vi "JWT Calculate Hash.vi"(0 "JSONWebToken in":refnum<class "JSONWebToken.lvclass">, 11 "error in (no error)":errorcluster) -> (4 "JSONWebToken out":refnum<class "JSONWebToken.lvclass">, 6 "signing input hash":string, 15 "error out":errorcluster)   [LabVIEW 2020, in "JSONWebToken.lvclass"]
doc: "If the algorithm in the token = \"RS256\", we know we need to generate the SHA-256 hash of the header and payload segments. This will reproduce the signing input hash. This hash should match the header+payload hash encrypted in the signature."
uses:
  JSONWebToken.lvclass
  JSONWebToken.lvclass/JSONWebToken.ctl
  <vilib>/security/Message Digest/API/Instances/Byte Array/SHA-256 Byte Array Checksum.vi
  <vilib>/security/Message Digest/API/NI_Message Digest API.lvlib
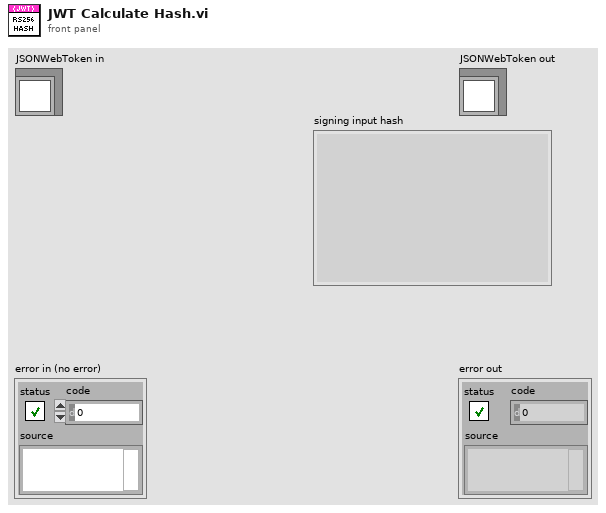
[diagram p1: front panel]
types:
  T1 = typedef "header.ctl" = cluster{"alg":string, "jku":string, "jwk":string, "kid":string, "x5u":string, "x5c":string, "x5t":string, "x5t#S256":string, "typ":string, "cty":string, "crit":string, "enc":string}
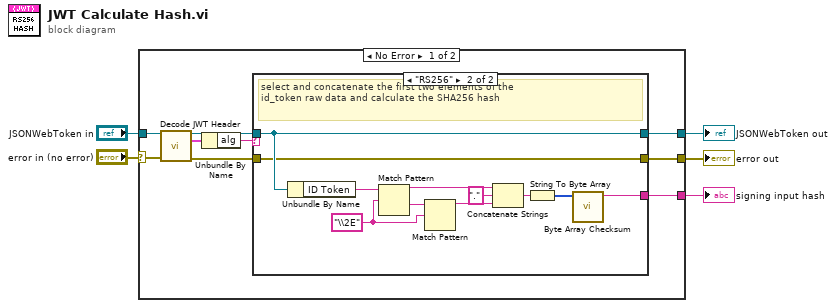
[diagram p0: block diagram]
diagram:
  n1 = case shown="No Error" "error in (no error)" {
    selector: "error in (no error)" -> [w11 w29]
    tunnel: [w7 w29] -> w4
    tunnel: [w6 w28] -> w2
    tunnel: "JSONWebToken in" -> [w13 w28]
    tunnel: [w14 _] -> w1
    frame No Error {
      n2 = call "Decode JWT Header.vi"("JSONWebToken in"=w13, "error in (no error)"=w11) -> ("JSONWebToken out"=w12:refnum<class "JSONWebToken.lvclass">, "JWT header"=w10:T1, "error out"=w8:errorcluster)  [unwired: 10 in, 1 out]
      n3 = Unbundle By Name(w10) -> ("alg"=w9:string)
      n4 = case shown="\"RS256\"" w9 {
        tunnel: [_ w18] -> w14
        tunnel: w12 -> [w15 w27]
        tunnel: w8 -> [w16 w26]
        tunnel: [w16 w26] -> w7
        tunnel: [w15 w27] -> w6
        frame "False", Default {
        }
        frame "RS256" {
          w23 = "\\2E" ("delimiter")
          # "select and concatenate the first two elements of the\nid_token raw data and calculate the SHA256 hash"
          n5 = Unbundle By Name(w27) -> ("ID Token"=w19:string)
          n6 = Match Pattern(string=w19, regular expression=w23) -> (before substring=w24:string, after substring=w25:string)  [unwired: 1 in, 2 out]
          n7 = Match Pattern(string=w25, regular expression=w23) -> (before substring=w22:string)  [unwired: 1 in, 3 out]
          n8 = Concatenate Strings(w24, "." ("string"), w22) -> (w20:string)
          n9 = String To Byte Array(string=w20) -> (unsigned byte array=w21:u8[])
          n10 = call-poly <vilib>:"Byte Array Checksum.vi"("buffer"=w21) -> ("digest"=w18:string)  [unwired: 10 in]
        }
      }
    }
    frame Error {
    }
  }
  "error out" <- w4
  "JSONWebToken out" <- w2
  "signing input hash" <- w1
